vi "08-12-中级计算器.vi"() -> ()   [LabVIEW 2025]
panel:
  out "过程显示":string
  out "操作临时值":string
  out "输入临时值":string
  out "结果":string
  out "输入2":string
  out "输入1":string
  in  "=":bool
  in  "清除":bool
  in  "/":bool
  in  "*":bool
  in  "-":bool
  in  "+":bool
  in  "小数点":bool
  in  "0":bool
  in  "±":bool
  in  "9":bool
  in  "8":bool
  in  "7":bool
  in  "6":bool
  in  "5":bool
  in  "4":bool
  in  "3":bool
  in  "2":bool
  in  "1":bool
  # "数字输入要放到输入临时值里"
  # "按下操作键之后，把输入临时值\n放到操作临时值里"
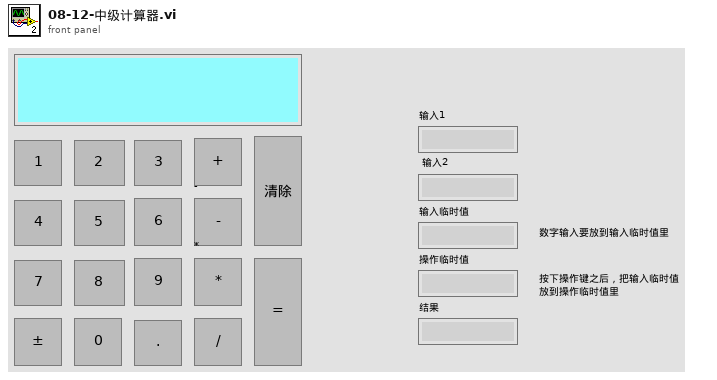
[diagram p1: front panel]
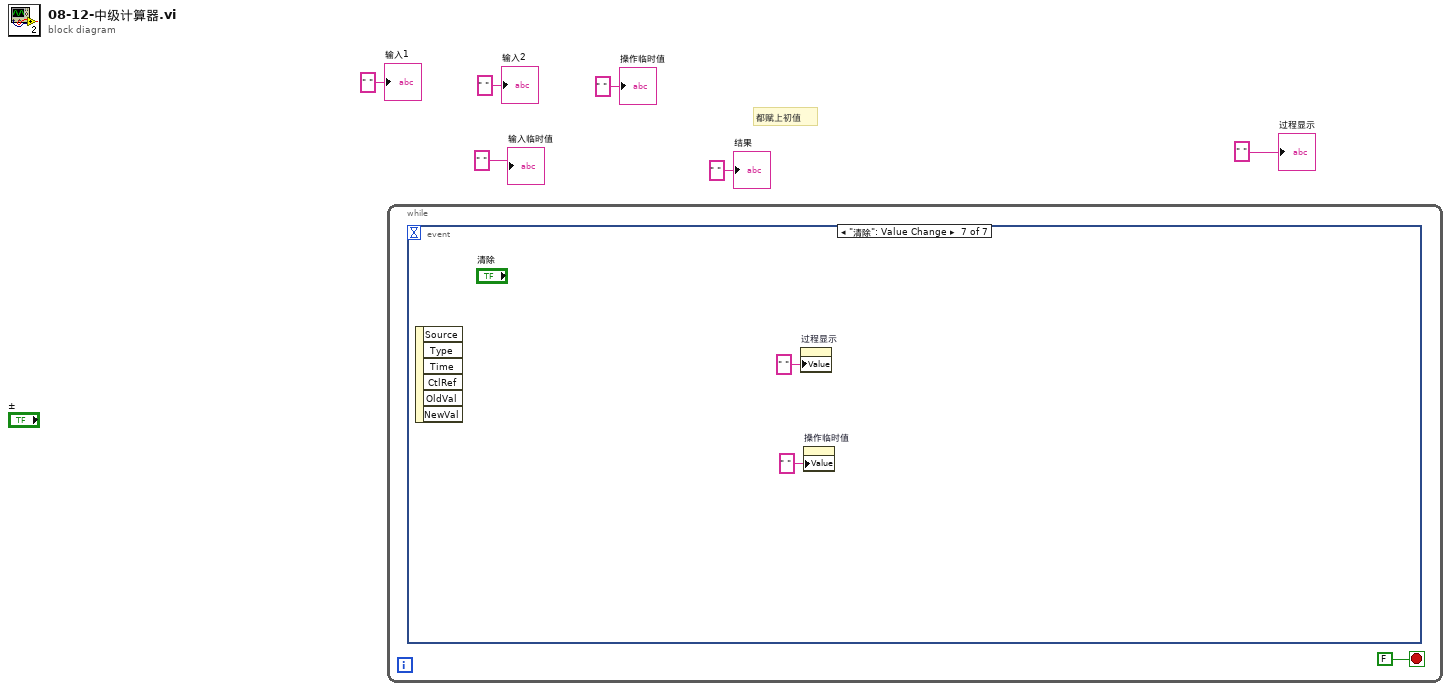
[diagram p0: block diagram]
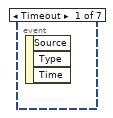
[diagram p2: hidden frame]
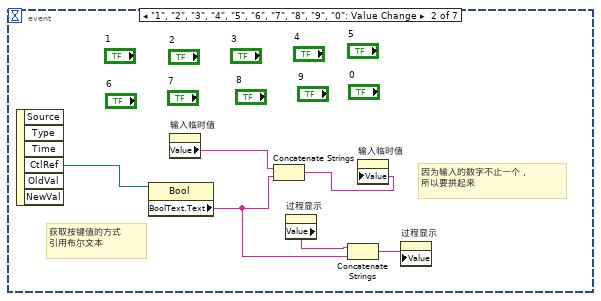
[diagram p3: hidden frame]
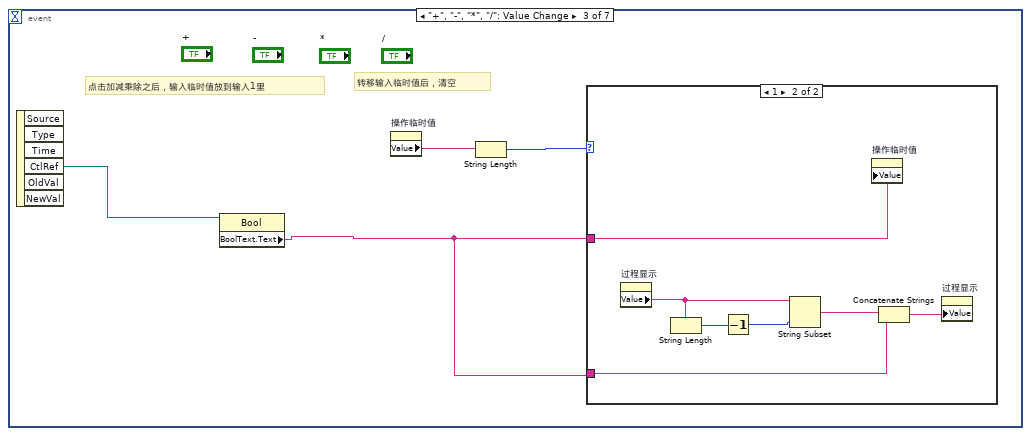
[diagram p4: hidden frame]
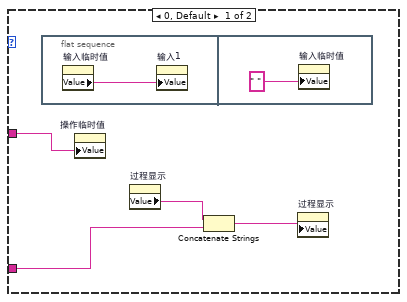
[diagram p5: hidden frame]
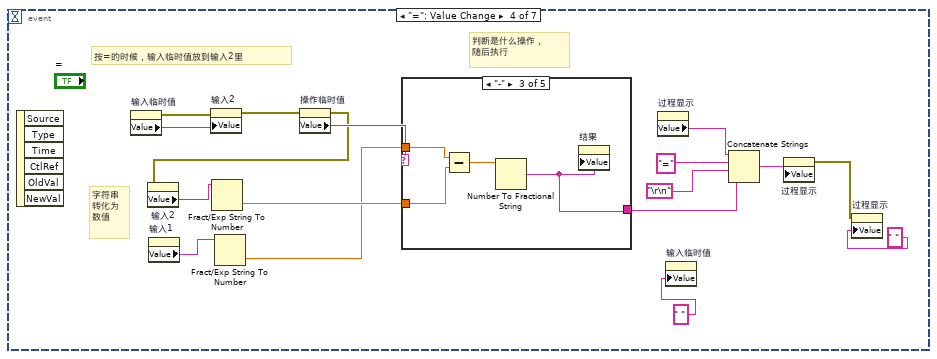
[diagram p6: hidden frame]
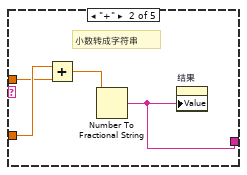
[diagram p8: hidden frame]
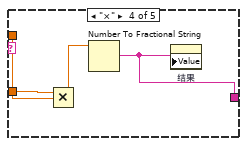
[diagram p9: hidden frame]
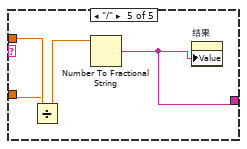
[diagram p10: hidden frame]
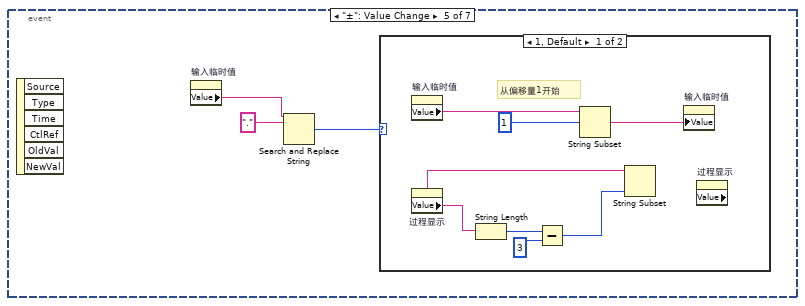
[diagram p11: hidden frame]
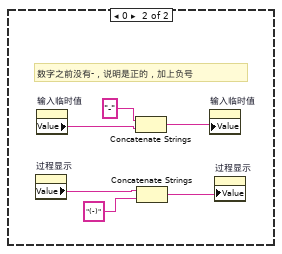
[diagram p12: hidden frame]
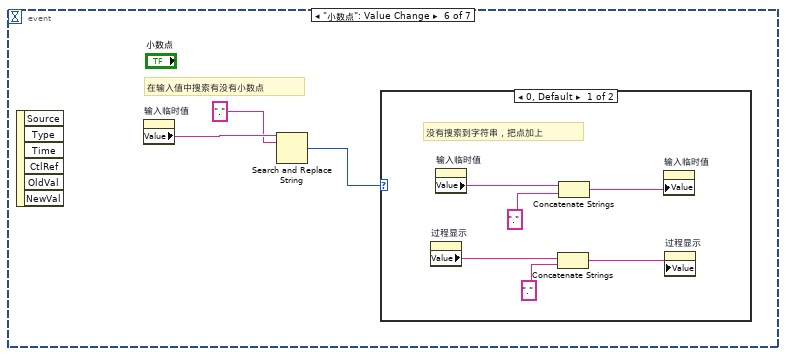
[diagram p13: hidden frame]
diagram:
  # "都赋上初值"
  n1 = while {
    stop <- FALSE stop-if-true
    n2 = event shown="[6] \"清除\": Value Change" {
      selector: _ -> [_ _ _ _ _ _ _]
      dyn-events: _ -> [_ _ _ _ _ _ _]
      timeout: _ -> [_ _ _ _ _ _ _]
      event Timeout {
        n3 = event-data() -> ()  [unwired: 1 in, 3 out]
      }
      event "1", "2", "3", "4", "5", "6", "7", "8", "9", "0": Value Change {
        # "因为输入的数字不止一个，\n所以要拼起来"
        # "获取按键值的方式\n引用布尔文本"
        n4 = event-data() -> ("CtlRef"=w13:refnum<vi>)  [unwired: 1 in, 5 out]
        n5 = property class="Bool"(reference=w13) -> ("BoolText.Text"=w8:string)  [unwired: 1 in, 2 out]
        n6 = property on="输入临时值" class="Str"() -> ("Value"=w12:string)  [unwired: 2 in, 2 out]
        n7 = Concatenate Strings(w12, w8) -> (w11:string)
        n8 = property on="过程显示" class="Str"() -> ("Value"=w9:string)  [unwired: 2 in, 2 out]
        n9 = Concatenate Strings(w9, w8) -> (w10:string)
        n10 = property on="输入临时值" class="Str"("Value"=w11) -> ()  [unwired: 2 in, 2 out]
        n11 = property on="过程显示" class="Str"("Value"=w10) -> ()  [unwired: 2 in, 2 out]
      }
      event "+", "-", "*", "/": Value Change {
        # "转移输入临时值后，清空"
        # "点击加减乘除之后，输入临时值放到输入1里"
        n12 = event-data() -> ("CtlRef"=w17:refnum<vi>)  [unwired: 1 in, 5 out]
        n13 = property class="Bool"(reference=w17) -> ("BoolText.Text"=w14:string)  [unwired: 1 in, 2 out]
        n14 = property on="操作临时值" class="Str"() -> ("Value"=w16:string)  [unwired: 2 in, 2 out]
        n15 = String Length(string=w16) -> (length=w15:i32)
        n16 = case shown="1" w15 {
          tunnel: w14 -> [w19 w30]
          tunnel: w14 -> [w18 w25]
          frame 0, Default {
            n17 = flat-sequence {
              frame #0 {
                n18 = property on="输入临时值" class="Str"() -> ("Value"=w22:string)  [unwired: 2 in, 2 out]
                n19 = property on="输入1" class="Str"("Value"=w22) -> ()  [unwired: 2 in, 2 out]
              }
              frame #1 {
                n20 = property on="输入临时值" class="Str"("Value"=" " ("输入临时值")) -> ()  [unwired: 2 in, 2 out]
              }
            }
            n21 = property on="操作临时值" class="Str"("Value"=w19) -> ()  [unwired: 2 in, 2 out]
            n22 = property on="过程显示" class="Str"() -> ("Value"=w20:string)  [unwired: 2 in, 2 out]
            n23 = Concatenate Strings(w20, w18) -> (w21:string)
            n24 = property on="过程显示" class="Str"("Value"=w21) -> ()  [unwired: 2 in, 2 out]
          }
          frame 1 {
            n25 = property on="过程显示" class="Str"() -> ("Value"=w27:string)  [unwired: 2 in, 2 out]
            n26 = String Length(string=w27) -> (length=w29:i32)
            n27 = Decrement(x=w29) -> (x-1=w28:i32)
            n28 = String Subset(string=w27, length (rest)=w28) -> (substring=w26:string)  [unwired: 1 in]
            n29 = property on="操作临时值" class="Str"("Value"=w30) -> ()  [unwired: 2 in, 2 out]
            n30 = Concatenate Strings(w26, w25) -> (w24:string)
            n31 = property on="过程显示" class="Str"("Value"=w24) -> ()  [unwired: 2 in, 2 out]
          }
        }
      }
      event "=": Value Change {
        # "字符串\n转化为\n数值"
        # "判断是什么操作，\n随后执行"
        # "按=的时候，输入临时值放到输入2里"
        n32 = event-data() -> ()  [unwired: 1 in, 6 out]
        n33 = property on="输入临时值" class="Str"() -> (error out=w45:errorcluster, "Value"=w47:string)  [unwired: 2 in, 1 out]
        n34 = property on="输入1" class="Str"() -> ("Value"=w44:string)  [unwired: 2 in, 2 out]
        n35 = property on="输入2" class="Str"(error in=w45, "Value"=w47) -> (error out=w42:errorcluster)  [unwired: 1 in, 1 out]
        n36 = Fract/Exp String To Number(string=w44) -> (number=w39:dbl)  [unwired: 3 in, 1 out]
        n37 = property on="操作临时值" class="Str"(error in=w42) -> (error out=w41:errorcluster, "Value"=w46:string)  [unwired: 1 in, 1 out]
        n38 = property on="输入2" class="Str"(error in=w41) -> ("Value"=w43:string)  [unwired: 1 in, 2 out]
        n39 = Fract/Exp String To Number(string=w43) -> (number=w40:dbl)  [unwired: 3 in, 1 out]
        n40 = case shown="\"-\"" w46 {
          tunnel: w40 -> [_ w50 w54 w59 w62]
          tunnel: w39 -> [_ w49 w55 w58 w63]
          tunnel: [_ w48 w52 w56 w60] -> w36
          frame "False", Default {
          }
          frame "+" {
            # "小数转成字符串"
            n41 = Add(x=w50, y=w49) -> (x+y=w51:dbl)
            n42 = Number To Fractional String(number=w51) -> (F-format string=w48:string)  [unwired: 3 in]
            n43 = property on="结果" class="Str"("Value"=w48) -> ()  [unwired: 2 in, 2 out]
          }
          frame "-" {
            n44 = Subtract(x=w55, y=w54) -> (x-y=w53:dbl)
            n45 = Number To Fractional String(number=w53) -> (F-format string=w52:string)  [unwired: 3 in]
            n46 = property on="结果" class="Str"("Value"=w52) -> ()  [unwired: 2 in, 2 out]
          }
          frame "×" {
            n47 = Multiply(x=w59, y=w58) -> (x*y=w57:dbl)
            n48 = Number To Fractional String(number=w57) -> (F-format string=w56:string)  [unwired: 3 in]
            n49 = property on="结果" class="Str"("Value"=w56) -> ()  [unwired: 2 in, 2 out]
          }
          frame "/" {
            n50 = Divide(x=w62, y=w63) -> (x/y=w61:dbl)
            n51 = Number To Fractional String(number=w61) -> (F-format string=w60:string)  [unwired: 3 in]
            n52 = property on="结果" class="Str"("Value"=w60) -> ()  [unwired: 2 in, 2 out]
          }
        }
        n53 = property on="过程显示" class="Str"() -> ("Value"=w35:string)  [unwired: 2 in, 2 out]
        n54 = property on="输入临时值" class="Str"("Value"=" " ("输入临时值")) -> ()  [unwired: 2 in, 2 out]
        n55 = Concatenate Strings(w35, "=" ("concatenated string"), "\r\n", w36) -> (w34:string)
        n56 = property on="过程显示" class="Str"("Value"=w34) -> (error out=w33:errorcluster)  [unwired: 2 in, 1 out]
        n57 = property on="过程显示" class="Str"(error in=w33, "Value"=" " ("过程显示")) -> ()  [unwired: 1 in, 2 out]
      }
      event "±": Value Change {
        n58 = event-data() -> ()  [unwired: 1 in, 6 out]
        n59 = property on="输入临时值" class="Str"() -> ("Value"=w66:string)  [unwired: 2 in, 2 out]
        n60 = Search and Replace String(input string=w66, replace string=".") -> (number of replacements=w64:i32)  [unwired: 6 in, 3 out]
        n61 = case shown="1, Default" w64 {
          frame 1, Default {
            # "从偏移量1开始"
            n62 = property on="输入临时值" class="Str"() -> ("Value"=w73:string)  [unwired: 2 in, 2 out]
            n63 = property on="过程显示" class="Str"() -> ("Value"=w70:string)  [unwired: 2 in, 2 out]
            n64 = String Length(string=w70) -> (length=w69:i32)
            n65 = Subtract(x=w69, y=3 ("x-y")) -> (x-y=w67:i32)
            n66 = String Subset(string=w73, offset (0)=1) -> (substring=w71:string)  [unwired: 1 in]
            n67 = String Subset(string=w70, length (rest)=w67) -> ()  [unwired: 1 in, 1 out]
            n68 = property on="输入临时值" class="Str"("Value"=w71) -> ()  [unwired: 2 in, 2 out]
            n69 = property on="过程显示" class="Str" props=["Value"]() -> ()  [unwired: 2 in, 3 out]
          }
          frame 0 {
            # "数字之前没有-，说明是正的，加上负号"
            n70 = property on="过程显示" class="Str"() -> ("Value"=w76:string)  [unwired: 2 in, 2 out]
            n71 = property on="输入临时值" class="Str"() -> ("Value"=w78:string)  [unwired: 2 in, 2 out]
            n72 = Concatenate Strings("-", w78) -> (w77:string)
            n73 = Concatenate Strings(w76, "(-)" ("string")) -> (w75:string)
            n74 = property on="输入临时值" class="Str"("Value"=w77) -> ()  [unwired: 2 in, 2 out]
            n75 = property on="过程显示" class="Str"("Value"=w75) -> ()  [unwired: 2 in, 2 out]
          }
        }
      }
      event "小数点": Value Change {
        # "在输入值中搜索有没有小数点"
        n76 = event-data() -> ()  [unwired: 1 in, 6 out]
        n77 = property on="输入临时值" class="Str"() -> ("Value"=w82:string)  [unwired: 2 in, 2 out]
        n78 = Search and Replace String(input string=w82, search string=".") -> (number of replacements=w80:i32)  [unwired: 6 in, 3 out]
        n79 = case shown="0, Default" w80 {
          frame 0, Default {
            # "没有搜索到字符串，把点加上"
            n80 = property on="过程显示" class="Str"() -> ("Value"=w84:string)  [unwired: 2 in, 2 out]
            n81 = property on="输入临时值" class="Str"() -> ("Value"=w88:string)  [unwired: 2 in, 2 out]
            n82 = Concatenate Strings(w84, "." ("concatenated string")) -> (w83:string)
            n83 = Concatenate Strings(w88, "." ("concatenated string")) -> (w86:string)
            n84 = property on="输入临时值" class="Str"("Value"=w86) -> ()  [unwired: 2 in, 2 out]
            n85 = property on="过程显示" class="Str"("Value"=w83) -> ()  [unwired: 2 in, 2 out]
          }
          frame 1 {
          }
        }
      }
      event "清除": Value Change {
        n86 = event-data() -> ()  [unwired: 1 in, 6 out]
        n87 = property on="过程显示" class="Str"("Value"=" " ("过程显示")) -> ()  [unwired: 2 in, 2 out]
        n88 = property on="操作临时值" class="Str"("Value"=" " ("操作临时值")) -> ()  [unwired: 2 in, 2 out]
      }
    }
  }
  "输入1" <- " " ("输入1")
  "输入2" <- " " ("输入2")
  "结果" <- " " ("结果")
  "输入临时值" <- " " ("输入临时值")
  "操作临时值" <- " " ("操作临时值")
  "过程显示" <- " " ("显示结果")
